vi "FTW-Regex-CapturingGroups.vi"(0 "Regex":refnum<class "FTW-Regex.lvclass">, 11 "error in":errorcluster) -> (4 "Regex out":refnum<class "FTW-Regex.lvclass">, 6 "Capture Groups":string[](array[string]), 15 "error out":errorcluster)   [LabVIEW 2013, in "FTW-Regex.lvclass"]
uses:
  FTW-Regex.lvclass
  FTW-Regex.lvclass/FTW-Regex.ctl
  error/FTW-ERR-ThrowError.vi
  error/FTW-ERR-NoErrorConstant.vi
  error/FTW-ERR-CallChain.vi
  string/FTW-STR-ReplaceWhitespace.vi
panel:
  # "Inputs"
  # "Outputs"
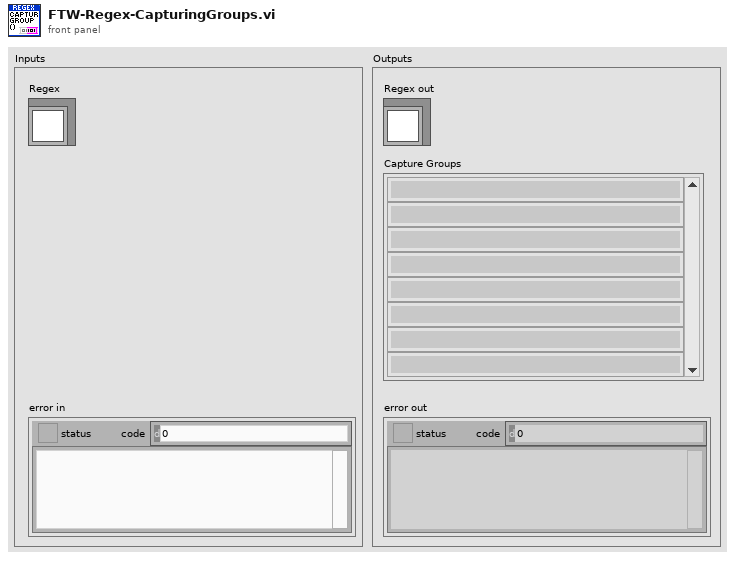
[diagram p1: front panel]
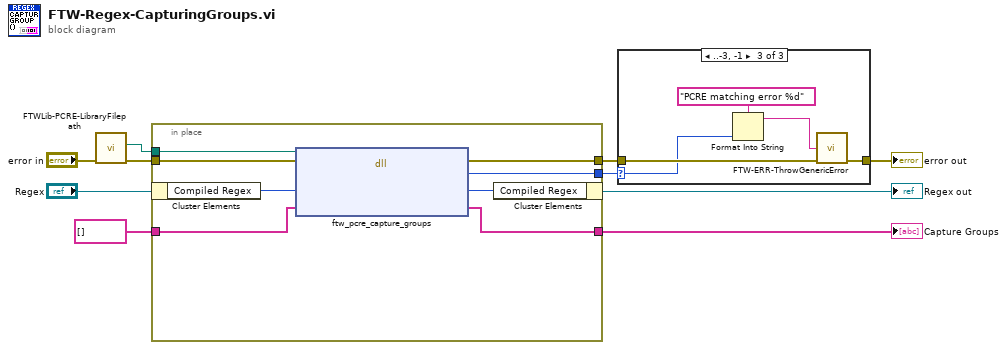
[diagram p0: block diagram]
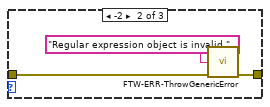
[diagram p3: hidden frame]
diagram:
  n1 = call "FTWLib-PCRE-LibraryFilepath.vi"("error in"="error in") -> ("error out"=w8:errorcluster, "PCRE Library Filepath"=w9:path)  [unwired: 8 in, 1 out]
  n2 = in-place {
    in-place-border: [w18] -> w3
    in-place-border: w9 -> [w17]
    in-place-border: w8 -> [w16]
    in-place-border: [w13] -> w5
    in-place-border: [w12] -> w2
    in-place-border: string[] [] -> [w11]
    n3 = in-place-cluster #1("Regex") -> ("Compiled Regex"=w15:u64)
    n4 = dll-call lib="?" fn="ftw_pcre_capture_groups"(path in=w17, error in=w16, "Compiled Regex"=w15, "Capture Groups"=w11) -> (error out=w18:errorcluster, "Return Value"=w13:i64, "Compiled Regex"=w14:u64, "Capture Groups"=w12:string[])  [unwired: 1 in, 1 out]
    n5 = in-place-cluster #1("Compiled Regex"=w14) -> (→"Regex out":refnum<class "FTW-Regex.lvclass">)
  }
  "Capture Groups" <- w2
  n6 = case shown="..-3, -1" w5 {
    selector: w5 -> [_ _ w25]
    tunnel: [w19 w21 w26] -> w4
    tunnel: w3 -> [w19 w22 w27]
    frame 0.. {
    }
    frame -2 {
      n7 = call "FTW-ERR-ThrowGenericError.vi"("Error Message"="Regular expression object is invalid.", "error in"=w22) -> ("error out"=w21:errorcluster)  [unwired: 13 in]
    }
    frame ..-3, -1 {
      n8 = Format Into String(format string="PCRE matching error %d" ("Error Message"), w25) -> (resulting string=w24:string)  [unwired: 2 in, 1 out]
      n9 = call "FTW-ERR-ThrowGenericError.vi"("Error Message"=w24, "error in"=w27) -> ("error out"=w26:errorcluster)  [unwired: 13 in]
    }
  }
  "error out" <- w4
